vi "Catalytic Methanation #2.vi"() -> ()   [LabVIEW 2017]
uses:
  <vilib>/addons/control/pid/pid.llb/PID Advanced (DBL).vi
  Halt S&THx.vi
  <vilib>/addons/control/pid/NI_PID_pid.lvlib
panel:
  out "Heater Power Confirmed":bool
  in  "Heater Switch":bool
  in  "CO2 Setpoint (SCCM)":dbl min=0.0 max=10.0 format="%.2f"
  in  "Temperature Setpoint (C)":dbl=20.0 min=0.0 max=325.0 format="%.1f"
  out "Reator Temperature (C)":dbl format="%.2f"
  out "Heater Output (%)":dbl(slide) scale=0.0..100.0
  in  "Manual Control Override (Temperature)":bool=TRUE
  in  "Set Manual Valve Heater Output (Temperature)":dbl(slide) scale=0.0..100.0
  in  "Reactor Pressure  Setpoint (psia)":dbl=18.4 min=0.0 max=30.0 format="%.1f"
  out "Reactor Pressure (psia)":dbl format="%.1f"
  out "Pressure Control Valve (%)":dbl(slide) scale=0.0..100.0
  in  "Manual Control Override (Pressure)":bool=TRUE
  in  "Set Manual Valve Position (Pressure)":dbl(slide)=50.0 scale=0.0..100.0
  in  "stop":bool
  in  "H2 Setpoint (SCCM)":dbl min=0.0 max=50.0 format="%.2f"
  in  "He Setpoint (SCCM)":dbl min=0.0 max=200.0 format="%.1f"
  out "CO2 Flowrate (SCCM)":dbl format="%.2f"
  out "H2 Flowrate (SCCM)":dbl format="%.2f"
  out "He Flowrate (SCCM)":dbl format="%.1f"
  in  "GC Sample Path":enum32{"Reactor Feed", "Reactor Exhaust"}(radio)=enum."Reactor Exhaust"
  in  "Kc (Heater)":dbl=1.0
  in  "Ti (Heater)":dbl=5.0 caption="(min)"
  in  "Td (Heater)":dbl caption="(min)"
  in  "Kc (Pressure)":dbl=-0.1
  in  "Ti (Pressure)":dbl=0.01
  in  "Td (Pressure)":dbl
  out "Data Point Count":i32
  in  "Specify Time between Data Points (sec)":dbl=1.0
  in  "Cancel Data Collection":bool
  in  "Specify number of data points":i16=1
  in  "Enable 4":bool
  out "Saving Data 4":bool
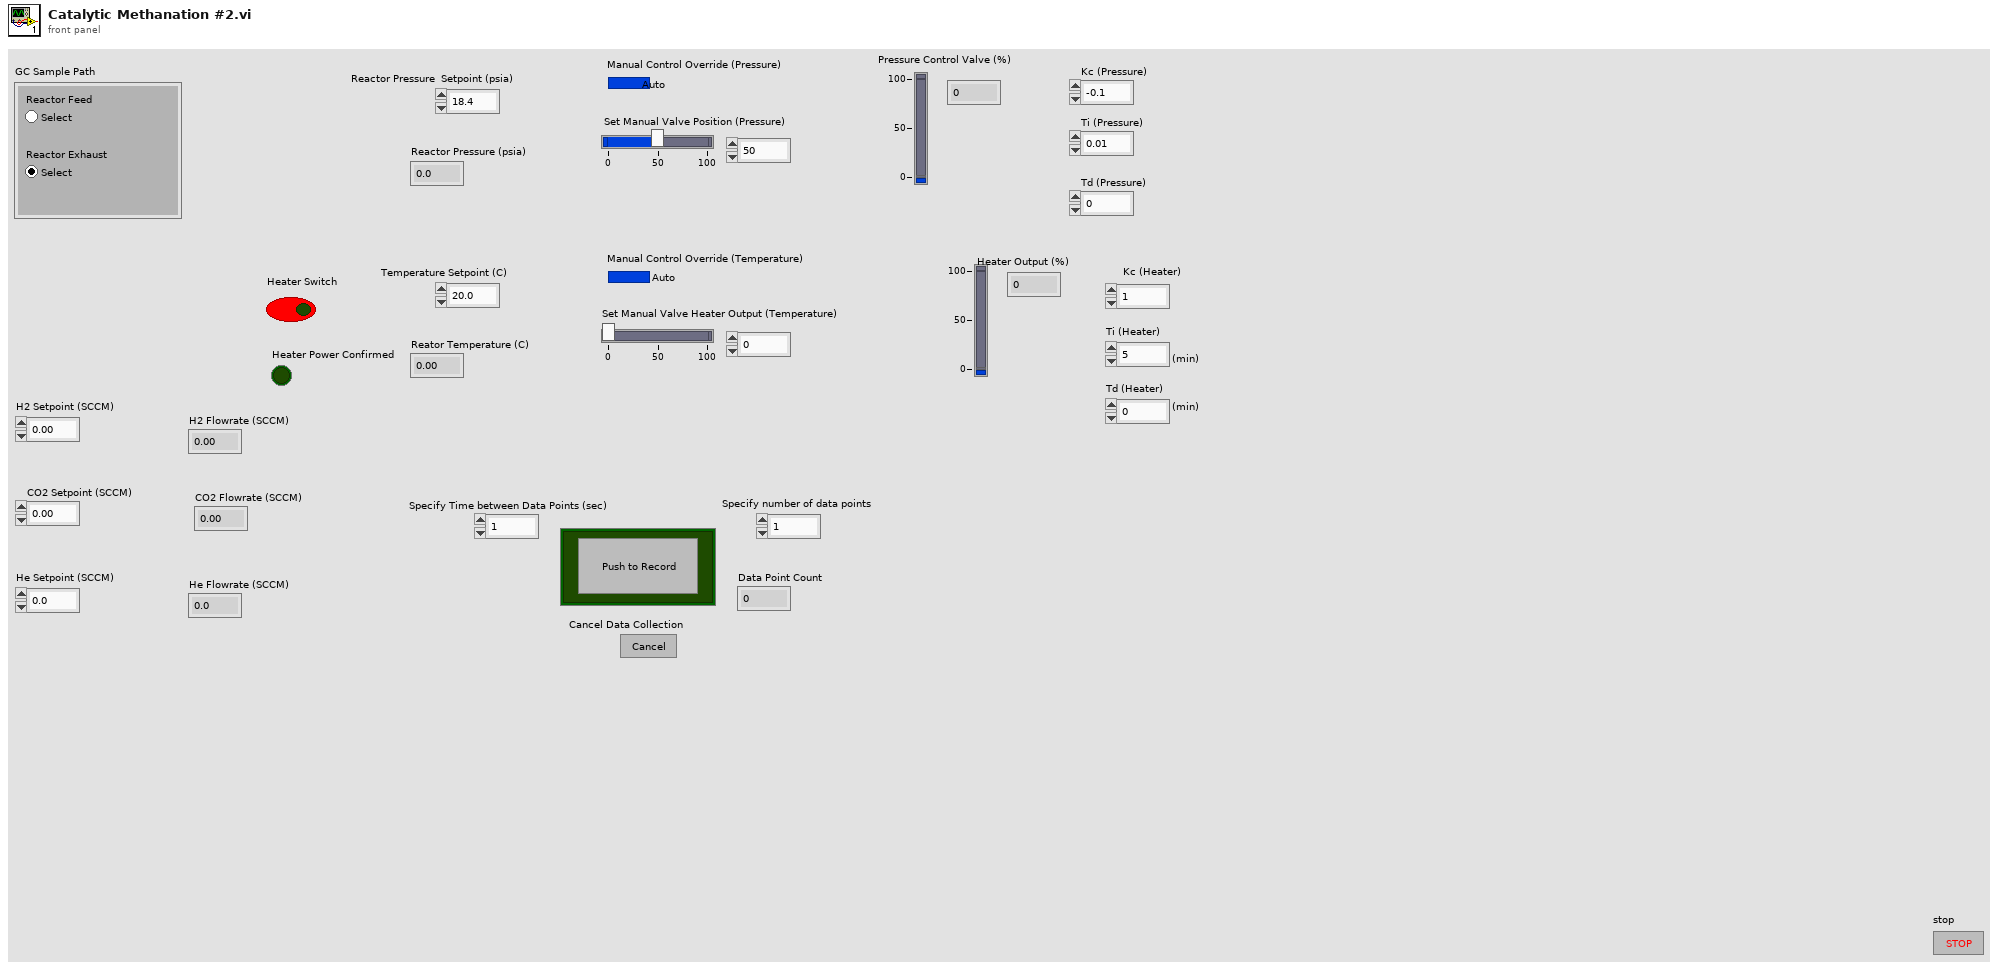
[diagram p1: front panel]
types:
  T1 = cluster{"Kc (Heater)":dbl, "Ti (Heater)":dbl, "Td (Heater)":dbl}
  T2 = cluster{"Kc (Pressure)":dbl, "Ti (Pressure)":dbl, "Td (Pressure)":dbl}
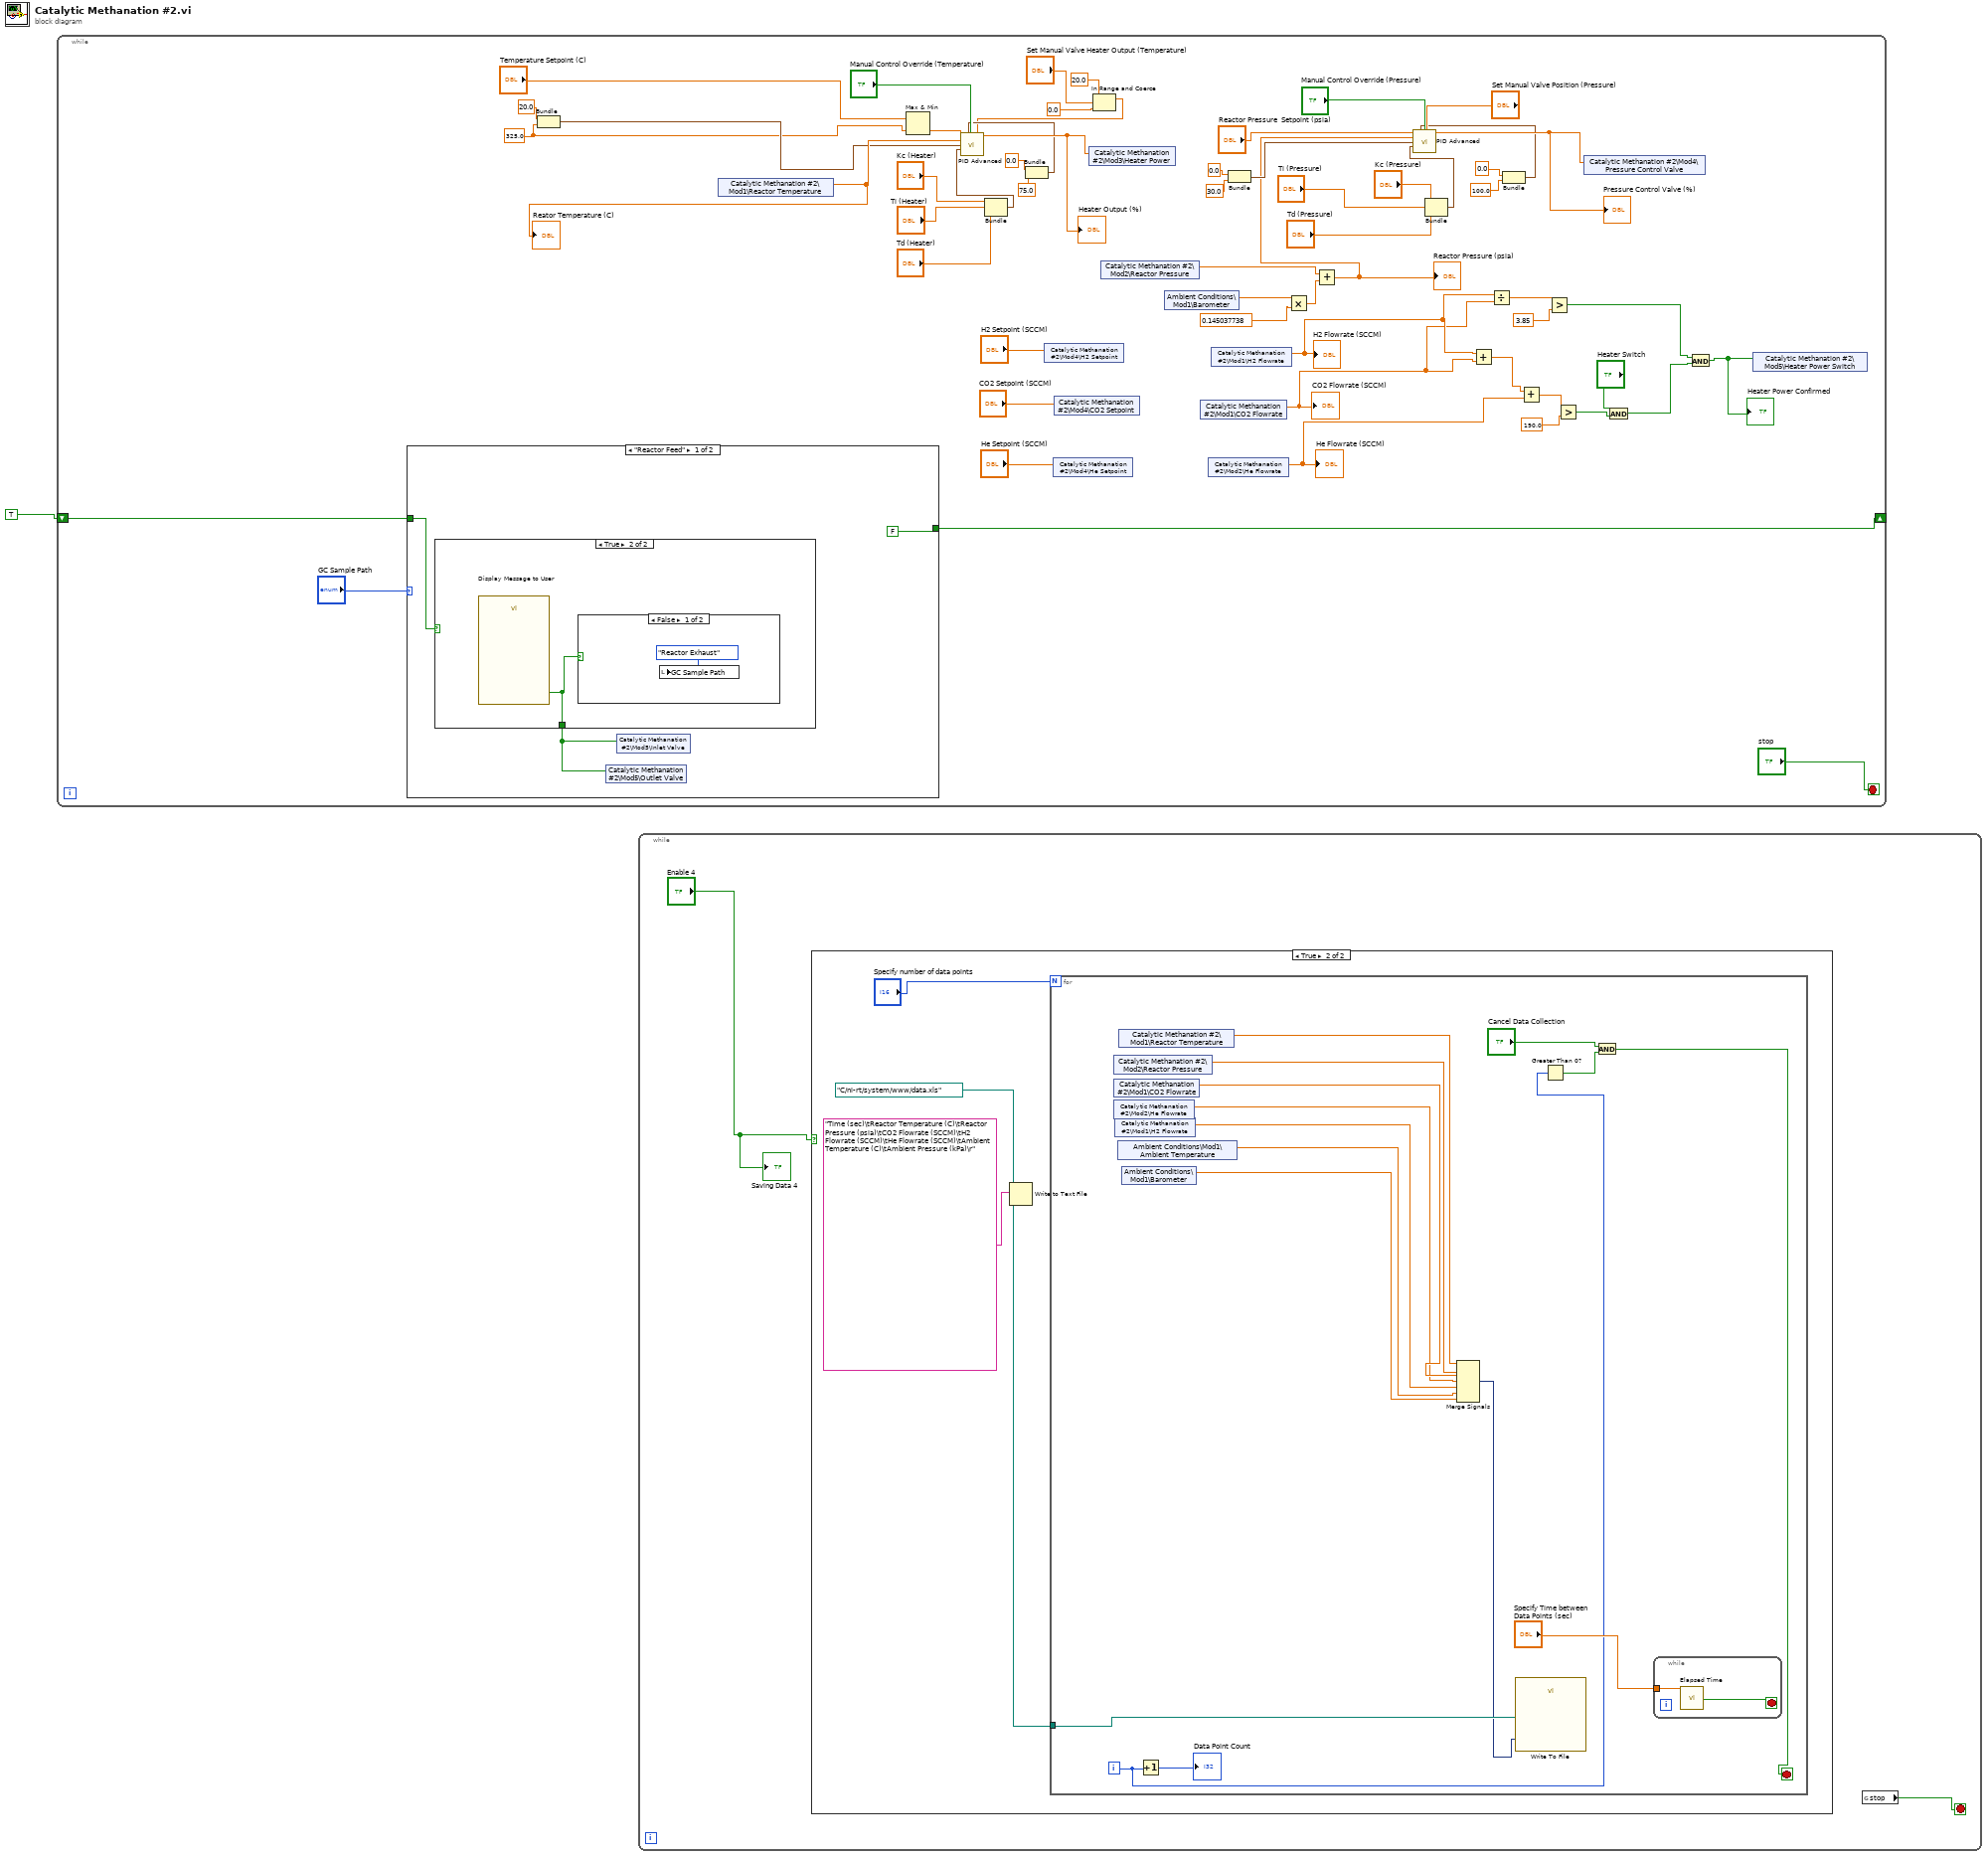
[diagram p0: block diagram]
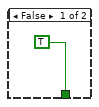
[diagram p2: hidden frame]
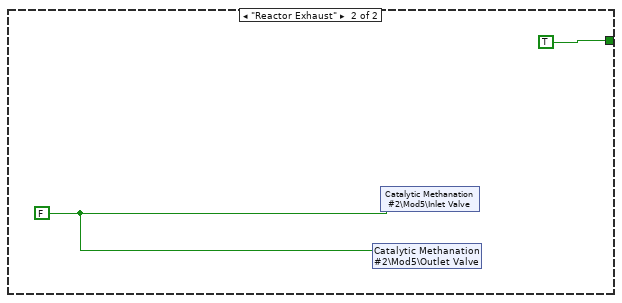
[diagram p4: hidden frame]
diagram:
  n1 = while {
    shift-right: [w9] -> _
    shift-left: TRUE -> [w10]
    stop <- "stop" stop-if-true
    w35 = 325.0
    n2 = case shown="\"Reactor Feed\"" "GC Sample Path" {
      tunnel: w10 -> [w62 _]
      tunnel: [FALSE TRUE] -> w9
      frame "Reactor Feed" {
        n3 = case shown="True" w62 {
          tunnel: [TRUE w64] -> w60
          frame False {
          }
          frame True {
            n4 = call "Display Message to User"() -> ("OK"=w64:bool)  [unwired: 10 in, 1 out]
            n5 = case shown="False" w64 {
              frame False {
                n6 = local write "GC Sample Path"(enum32{"Reactor Feed", "Reactor Exhaust"}."Reactor Exhaust" ("GC Sample Path")) -> ()
              }
              frame True {
              }
            }
          }
        }
        n7 = shared-variable "Catalytic Methanation #2\\Mod5\\Outlet Valve"(w60) -> ()  [unwired: 1 in, 1 out]
        n8 = shared-variable "Catalytic Methanation #2\\Mod5\\Inlet Valve"(w60) -> ()  [unwired: 1 in, 1 out]
      }
      frame "Reactor Exhaust" {
        w67 = FALSE
        n9 = shared-variable "Catalytic Methanation #2\\Mod5\\Outlet Valve"(w67) -> ()  [unwired: 1 in, 1 out]
        n10 = shared-variable "Catalytic Methanation #2\\Mod5\\Inlet Valve"(w67) -> ()  [unwired: 1 in, 1 out]
      }
    }
    n11 = Bundle(20.0, w35) -> (w37:cluster{dbl, dbl})  [unwired: 1 in]
    n12 = shared-variable "Catalytic Methanation #2\\Mod1\\Reactor Temperature"() -> (w46:dbl)  [unwired: 1 in, 1 out]
    "Reator Temperature (C)" <- w46
    n13 = Max & Min(x="Temperature Setpoint (C)", y=w35) -> (min(x,y)=w27:dbl)  [unwired: 1 out]
    n14 = Bundle("Kc (Heater)"="Kc (Heater)", "Ti (Heater)"="Ti (Heater)", "Td (Heater)"="Td (Heater)") -> (w55:T1)  [unwired: 1 in]
    n15 = Bundle(0.0, 75.0) -> (w39:cluster{dbl, dbl})  [unwired: 1 in]
    n16 = shared-variable "Catalytic Methanation #2\\Mod4\\H2 Setpoint"("H2 Setpoint (SCCM)") -> ()  [unwired: 1 in, 1 out]
    n17 = shared-variable "Catalytic Methanation #2\\Mod4\\He Setpoint"("He Setpoint (SCCM)") -> ()  [unwired: 1 in, 1 out]
    n18 = shared-variable "Catalytic Methanation #2\\Mod4\\CO2 Setpoint"("CO2 Setpoint (SCCM)") -> ()  [unwired: 1 in, 1 out]
    n19 = In Range and Coerce(upper limit=20.0, x="Set Manual Valve Heater Output (Temperature)", lower limit=0.0) -> (coerced(x)=w25:dbl)  [unwired: 1 out]
    n20 = call-poly <vilib>:"PID Advanced.vi"("setpoint"=w27, "output range"=w39, "auto? (T)"="Manual Control Override (Temperature)", "manual control"=w25, "process variable"=w46, "setpoint range"=w37, "PID gains"=w55) -> ("output"=w48:dbl)  [unwired: 7 in, 1 out]
    "Heater Output (%)" <- w48
    n21 = shared-variable "Catalytic Methanation #2\\Mod3\\Heater Power"(w48) -> ()  [unwired: 1 in, 1 out]
    n22 = shared-variable "Catalytic Methanation #2\\Mod2\\Reactor Pressure"() -> (w17:dbl)  [unwired: 1 in, 1 out]
    n23 = shared-variable "Ambient Conditions\\Mod1\\Barometer"() -> (w21:dbl)  [unwired: 1 in, 1 out]
    n24 = shared-variable "Catalytic Methanation #2\\Mod1\\CO2 Flowrate"() -> (w7:dbl)  [unwired: 1 in, 1 out]
    "CO2 Flowrate (SCCM)" <- w7
    n25 = shared-variable "Catalytic Methanation #2\\Mod2\\He Flowrate"() -> (w15:dbl)  [unwired: 1 in, 1 out]
    "He Flowrate (SCCM)" <- w15
    n26 = shared-variable "Catalytic Methanation #2\\Mod1\\H2 Flowrate"() -> (w8:dbl)  [unwired: 1 in, 1 out]
    "H2 Flowrate (SCCM)" <- w8
    n27 = Bundle(0.0, 30.0) -> (w33:cluster{dbl, dbl})  [unwired: 1 in]
    n28 = Multiply(x=w21, y=0.145037738) -> (x*y=w19:dbl)
    n29 = Add(x=w17, y=w19) -> (x+y=w18:dbl)
    "Reactor Pressure (psia)" <- w18
    n30 = Bundle("Kc (Pressure)"="Kc (Pressure)", "Ti (Pressure)"="Ti (Pressure)", "Td (Pressure)"="Td (Pressure)") -> (w56:T2)  [unwired: 1 in]
    n31 = Add(x=w8, y=w7) -> (x+y=w16:dbl)
    n32 = Divide(x=w8, y=w7) -> (x/y=w6:dbl)
    n33 = Bundle(0.0, 100.0) -> (w30:cluster{dbl, dbl})  [unwired: 1 in]
    n34 = call-poly <vilib>:"PID Advanced.vi"("setpoint"="Reactor Pressure  Setpoint (psia)", "output range"=w30, "auto? (T)"="Manual Control Override (Pressure)", "manual control"="Set Manual Valve Position (Pressure)", "process variable"=w18, "setpoint range"=w33, "PID gains"=w56) -> ("output"=w59:dbl)  [unwired: 7 in, 1 out]
    "Pressure Control Valve (%)" <- w59
    n35 = Add(x=w16, y=w15) -> (x+y=w14:dbl)
    n36 = Greater?(x=w6, y=3.85) -> (0:w4:bool)
    n37 = Greater?(x=w14, y=190.0) -> (0:w11:bool)
    n38 = shared-variable "Catalytic Methanation #2\\Mod4\\Pressure Control Valve"(w59) -> ()  [unwired: 1 in, 1 out]
    n39 = And(x="Heater Switch", y=w11) -> (x .and. y?=w3:bool)
    n40 = And(x=w4, y=w3) -> (x .and. y?=w2:bool)
    "Heater Power Confirmed" <- w2
    n41 = shared-variable "Catalytic Methanation #2\\Mod5\\Heater Power Switch"(w2) -> ()  [unwired: 1 in, 1 out]
  }
  n42 = while {
    stop <- w68 stop-if-true
    n43 = case shown="True" "Enable 4" {
      frame False {
      }
      frame True {
        w71 = path "C:/ni-rt/system/www/data.xls" ("Filename")
        n44 = Write to Text File(file (use dialog)=w71, text="Time (sec)\tReactor Temperature (C)\tReactor Pressure (psia)\tCO2 Flowrate (SCCM)\tH2 Flowrate (SCCM)\tHe Flowrate (SCCM)\tAmbient Temperature (C)\tAmbient Pressure (kPa)\r") -> ()  [unwired: 2 in, 3 out]
        n45 = for {
          N: "Specify number of data points" -> [_]
          tunnel: w71 -> [w87]
          i -> [w81]
          stop <- w78 stop-if-true
          n46 = shared-variable "Catalytic Methanation #2\\Mod1\\CO2 Flowrate"() -> (w84:dbl)  [unwired: 1 in, 1 out]
          n47 = shared-variable "Catalytic Methanation #2\\Mod2\\Reactor Pressure"() -> (w85:dbl)  [unwired: 1 in, 1 out]
          n48 = shared-variable "Catalytic Methanation #2\\Mod2\\He Flowrate"() -> (w77:dbl)  [unwired: 1 in, 1 out]
          n49 = shared-variable "Catalytic Methanation #2\\Mod1\\H2 Flowrate"() -> (w76:dbl)  [unwired: 1 in, 1 out]
          n50 = shared-variable "Ambient Conditions\\Mod1\\Ambient Temperature"() -> (w74:dbl)  [unwired: 1 in, 1 out]
          n51 = shared-variable "Catalytic Methanation #2\\Mod1\\Reactor Temperature"() -> (w75:dbl)  [unwired: 1 in, 1 out]
          n52 = shared-variable "Ambient Conditions\\Mod1\\Barometer"() -> (w73:dbl)  [unwired: 1 in, 1 out]
          n53 = Increment(x=w81) -> (x+1=→"Data Point Count":i32)
          n54 = Merge Signals(w75, w85, w84, w77, w76, w74, w73) -> (w83:dynamicdata)
          n55 = call "Write To File"("Signals"=w83, "Filename"=w87) -> ()  [unwired: 15 in, 3 out]
          n56 = Greater Than 0?(x=w81) -> (x > 0?=w79:bool)
          n57 = And(x="Cancel Data Collection", y=w79) -> (x .and. y?=w78:bool)
          n58 = while {
            tunnel: "Specify Time between Data Points (sec)" -> [w88]
            stop <- w89 stop-if-true
            n59 = call "Elapsed Time"("Time Target (s)"=w88) -> ("Time has Elapsed"=w89:bool)  [unwired: 11 in, 7 out]
          }
        }
      }
    }
    n60 = global read "Halt S&THx.vi" "stop"() -> (w68:bool)
    "Saving Data 4" <- "Enable 4"
  }
